vi "Evaluate Test Results.vi"(8 "error in (no error)":errorcluster, 9 "Test Info":T1, 10 "Test Config":T2, 11 "Test Results":T8) -> (0 "error out":errorcluster, 1 "Summary Out":string[][](array[string]), 2 "Vacuum Results":string[][](array[string]), 3 "Helium Results":string[][](array[string]), 5 "Report Name":string)   [LabVIEW 2014]
uses:
  Tests/Controls/Test Results.ctl
  Tests/Controls/Step Result.ctl
  Tests/Controls/Test Information.ctl
  Tests/Controls/Vacuum Test.ctl
  Tests/Controls/Test Timing.ctl
  Tests/Controls/Vaccum Thresholds.ctl
  Tests/Controls/Helium Test.ctl
  Tests/Controls/Helium Thresholds.ctl
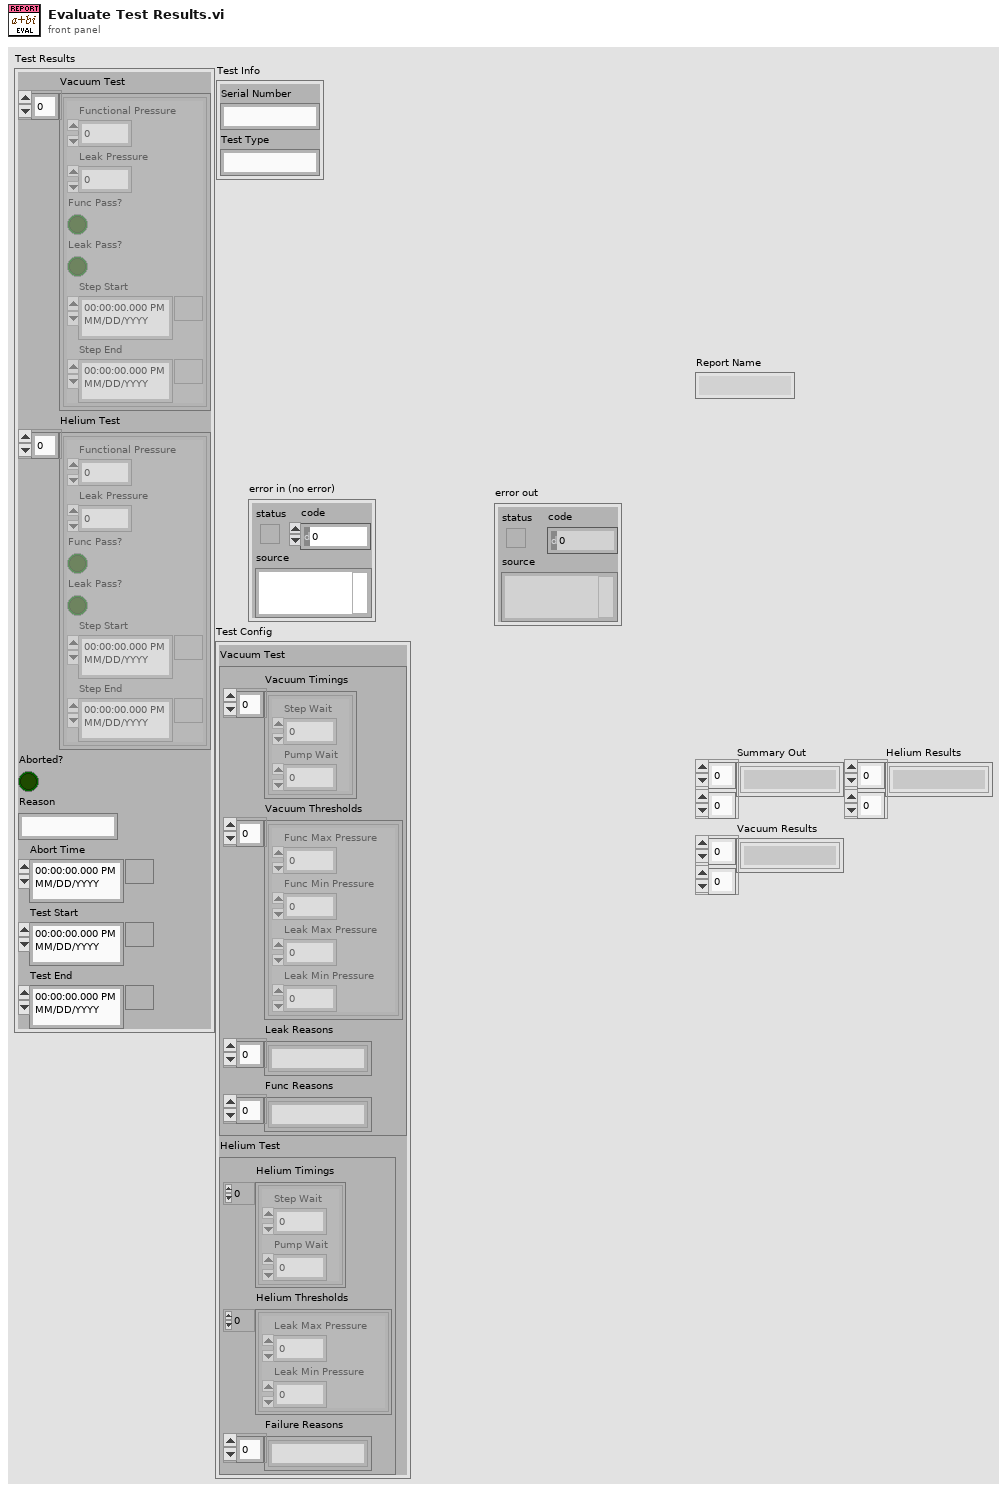
[diagram p1: front panel]
types:
  T1 = cluster{"Serial Number":string, "Test Type":string}
  T2 = typedef "Test Information.ctl" = cluster{"Vacuum Test":T3, "Helium Test":T6}
  T3 = typedef "Vacuum Test.ctl" = cluster{"Vacuum Timings":T4[], "Vacuum Thresholds":T5[], "Leak Reasons":string[], "Func Reasons":string[]}
  T4 = typedef "Test Timing.ctl" = cluster{"Step Wait":dbl, "Pump Wait":dbl}
  T5 = typedef "Vaccum Thresholds.ctl" = cluster{"Func Max Pressure":dbl, "Func Min Pressure":dbl, "Leak Max Pressure":dbl, "Leak Min Pressure":dbl}
  T6 = typedef "Helium Test.ctl" = cluster{"Helium Timings":T4[], "Helium Thresholds":T7[], "Failure Reasons":string[]}
  T7 = typedef "Helium Thresholds.ctl" = cluster{"Leak Max Pressure":dbl, "Leak Min Pressure":dbl}
  T8 = typedef "Test Results.ctl" = cluster{"Vacuum Test":T9[], "Helium Test":T9[], "Aborted?":bool, "Reason":string, "Abort Time":timestamp, "Test Start":timestamp, "Test End":timestamp}
  T9 = typedef "Step Result.ctl" = cluster{"Functional Pressure":dbl, "Leak Pressure":dbl, "Func Pass?":bool, "Leak Pass?":bool, "Step Start":timestamp, "Step End":timestamp}
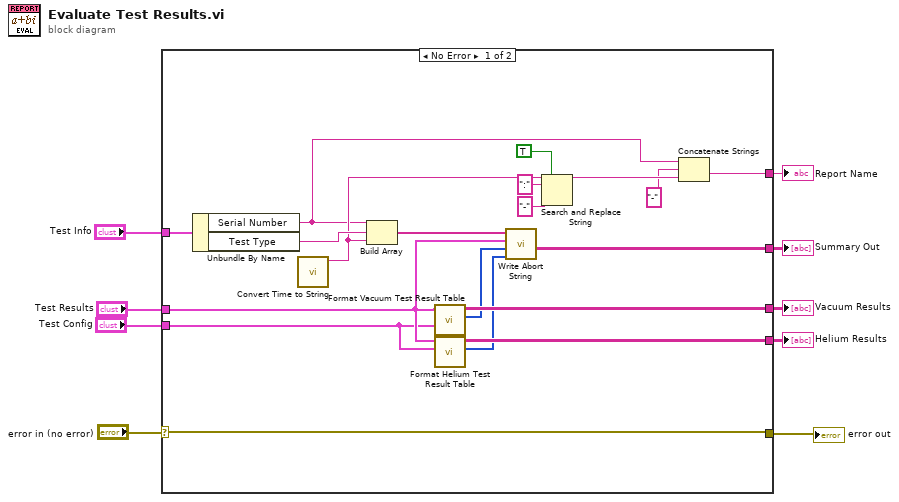
[diagram p0: block diagram]
diagram:
  n1 = case shown="No Error" "error in (no error)" {
    selector: "error in (no error)" -> [w25 w29]
    tunnel: [w25 w29] -> w9
    tunnel: "Test Results" -> [w20 _]
    tunnel: "Test Config" -> [w19 _]
    tunnel: "Test Info" -> [w26 _]
    tunnel: [w24 _] -> w3
    tunnel: [w23 _] -> w2
    tunnel: [w18 _] -> w4
    tunnel: [w12 _] -> w1
    frame No Error {
      n2 = Unbundle By Name(w26) -> ("Serial Number"=w10:string, "Test Type"=w28:string)
      n3 = call "Convert Time to String.vi"() -> ("date/time string"=w17:string)  [unwired: 11 in]
      n4 = Build Array(w10, w28, w17) -> (w27:string[])
      n5 = call "Format Vacuum Test Result Table.vi"("Test Config"=w19, "Test Results"=w20) -> ("Failure Indexes"=w22:i32[], "Vacuum Results"=w24:string[][])  [unwired: 8 in]
      n6 = call "Format Helium Test Result Table.vi"("Test Config"=w19, "Test Results"=w20) -> ("Failure Indexes"=w21:i32[], "Helium Results"=w23:string[][])  [unwired: 8 in]
      n7 = call "Write Abort String.vi"("Helium Fail"=w21, "Vacuum Fail"=w22, "Test Results"=w20, "Summary In"=w27) -> ("Summary Out"=w18:string[][])  [unwired: 7 in]
      n8 = Search and Replace String(replace all?=TRUE ("replace all? (F)"), input string=w17, search string=":", replace string="-" ("replace string (\"\")")) -> (result string=w13:string)  [unwired: 4 in, 3 out]
      n9 = Concatenate Strings(w10, "-" ("string"), w13) -> (w12:string)
    }
    frame Error {
    }
  }
  "error out" <- w9
  "Summary Out" <- w4
  "Vacuum Results" <- w3
  "Helium Results" <- w2
  "Report Name" <- w1
